vi "SplineParam_Spline_T0_T1.vi"(9 "T1":dbl, 10 "T0":dbl, 11 "inputSPLINE":T5) -> (0 "error out":errorcluster, 3 "outputPOSEwCURVATURE":T1[](array[typedef]))   [LabVIEW 2019, in "Trajectory_Library.lvlib"]
doc: "Parameterizes the spline. This method breaks up the spline into various arcs until their dx, dy, and dtheta are within specific tolerances.\n\nParameters:\n - InputSpline - The spline to parameterize.\n - T0 - Starting internal spline parameter. It is recommended to use 0.0.\n - T1 - Ending internal spline parameter. It is recommended to use 1.0.\n\nReturns:\n - OutputPoseWCurvature - A list of poses and curvatures that represents various points on the spline.\n - Error Out - Returned error cluster"
uses:
  Trajectory_Library.lvlib
  SPLINE.ctl
  <vilib>/Analysis/Matrix/Datatypes/RealMatrix.ctl
  POSEwCURVATURE.ctl
  POSE2D.ctl
  TRANSLATION2D.ctl
  ROTATION2D.ctl
  PARAM_STACK.ctl
  PARAM_STACK_ITEM.ctl
  <vilib>/Analysis/Matrix/NI_Matrix.lvlib
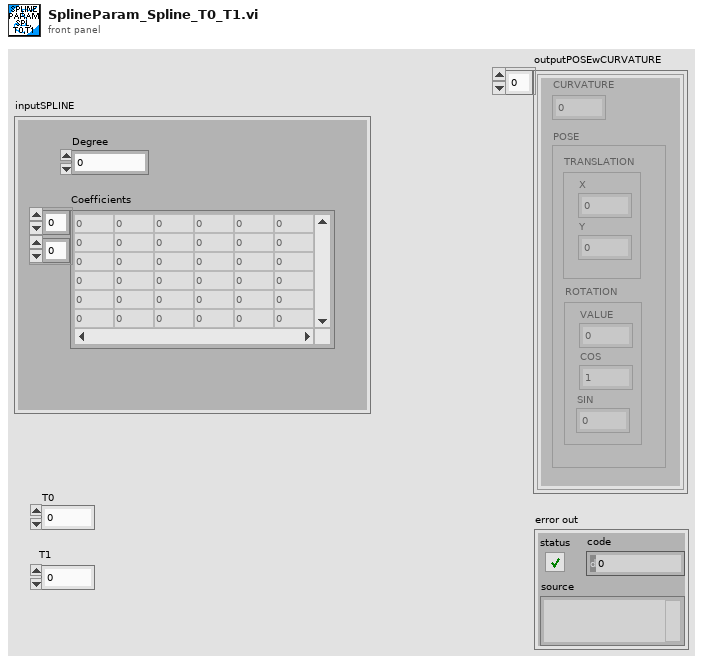
[diagram p1: front panel]
types:
  T1 = typedef "Trajectory_Library.lvlib/POSEwCURVATURE.ctl" = cluster{"CURVATURE":dbl, "POSE":T2}
  T2 = typedef "Trajectory_Library.lvlib/POSE2D.ctl" = cluster{"TRANSLATION":T3, "ROTATION":T4}
  T3 = typedef "Trajectory_Library.lvlib/TRANSLATION2D.ctl" = cluster{"X":dbl, "Y":dbl}
  T4 = typedef "Trajectory_Library.lvlib/ROTATION2D.ctl" = cluster{"VALUE":dbl, "COS":dbl, "SIN":dbl}
  T5 = typedef "Trajectory_Library.lvlib/SPLINE.ctl" = cluster{"Degree":i32, "Coefficients":T6}
  T6 = typedef "NI_Matrix.lvlib/RealMatrix.ctl" = dbl[][]
  T7 = typedef "Trajectory_Library.lvlib/PARAM_STACK.ctl" = cluster{"StackItems":i32, "Stack":T8[]}
  T8 = typedef "Trajectory_Library.lvlib/PARAM_STACK_ITEM.ctl" = cluster{"T0":dbl, "T1":dbl}
  T9 = typedef "Trajectory_Library.lvlib/TWIST2D.ctl" = cluster{"dX":dbl, "dY":dbl, "dTHETA":dbl}
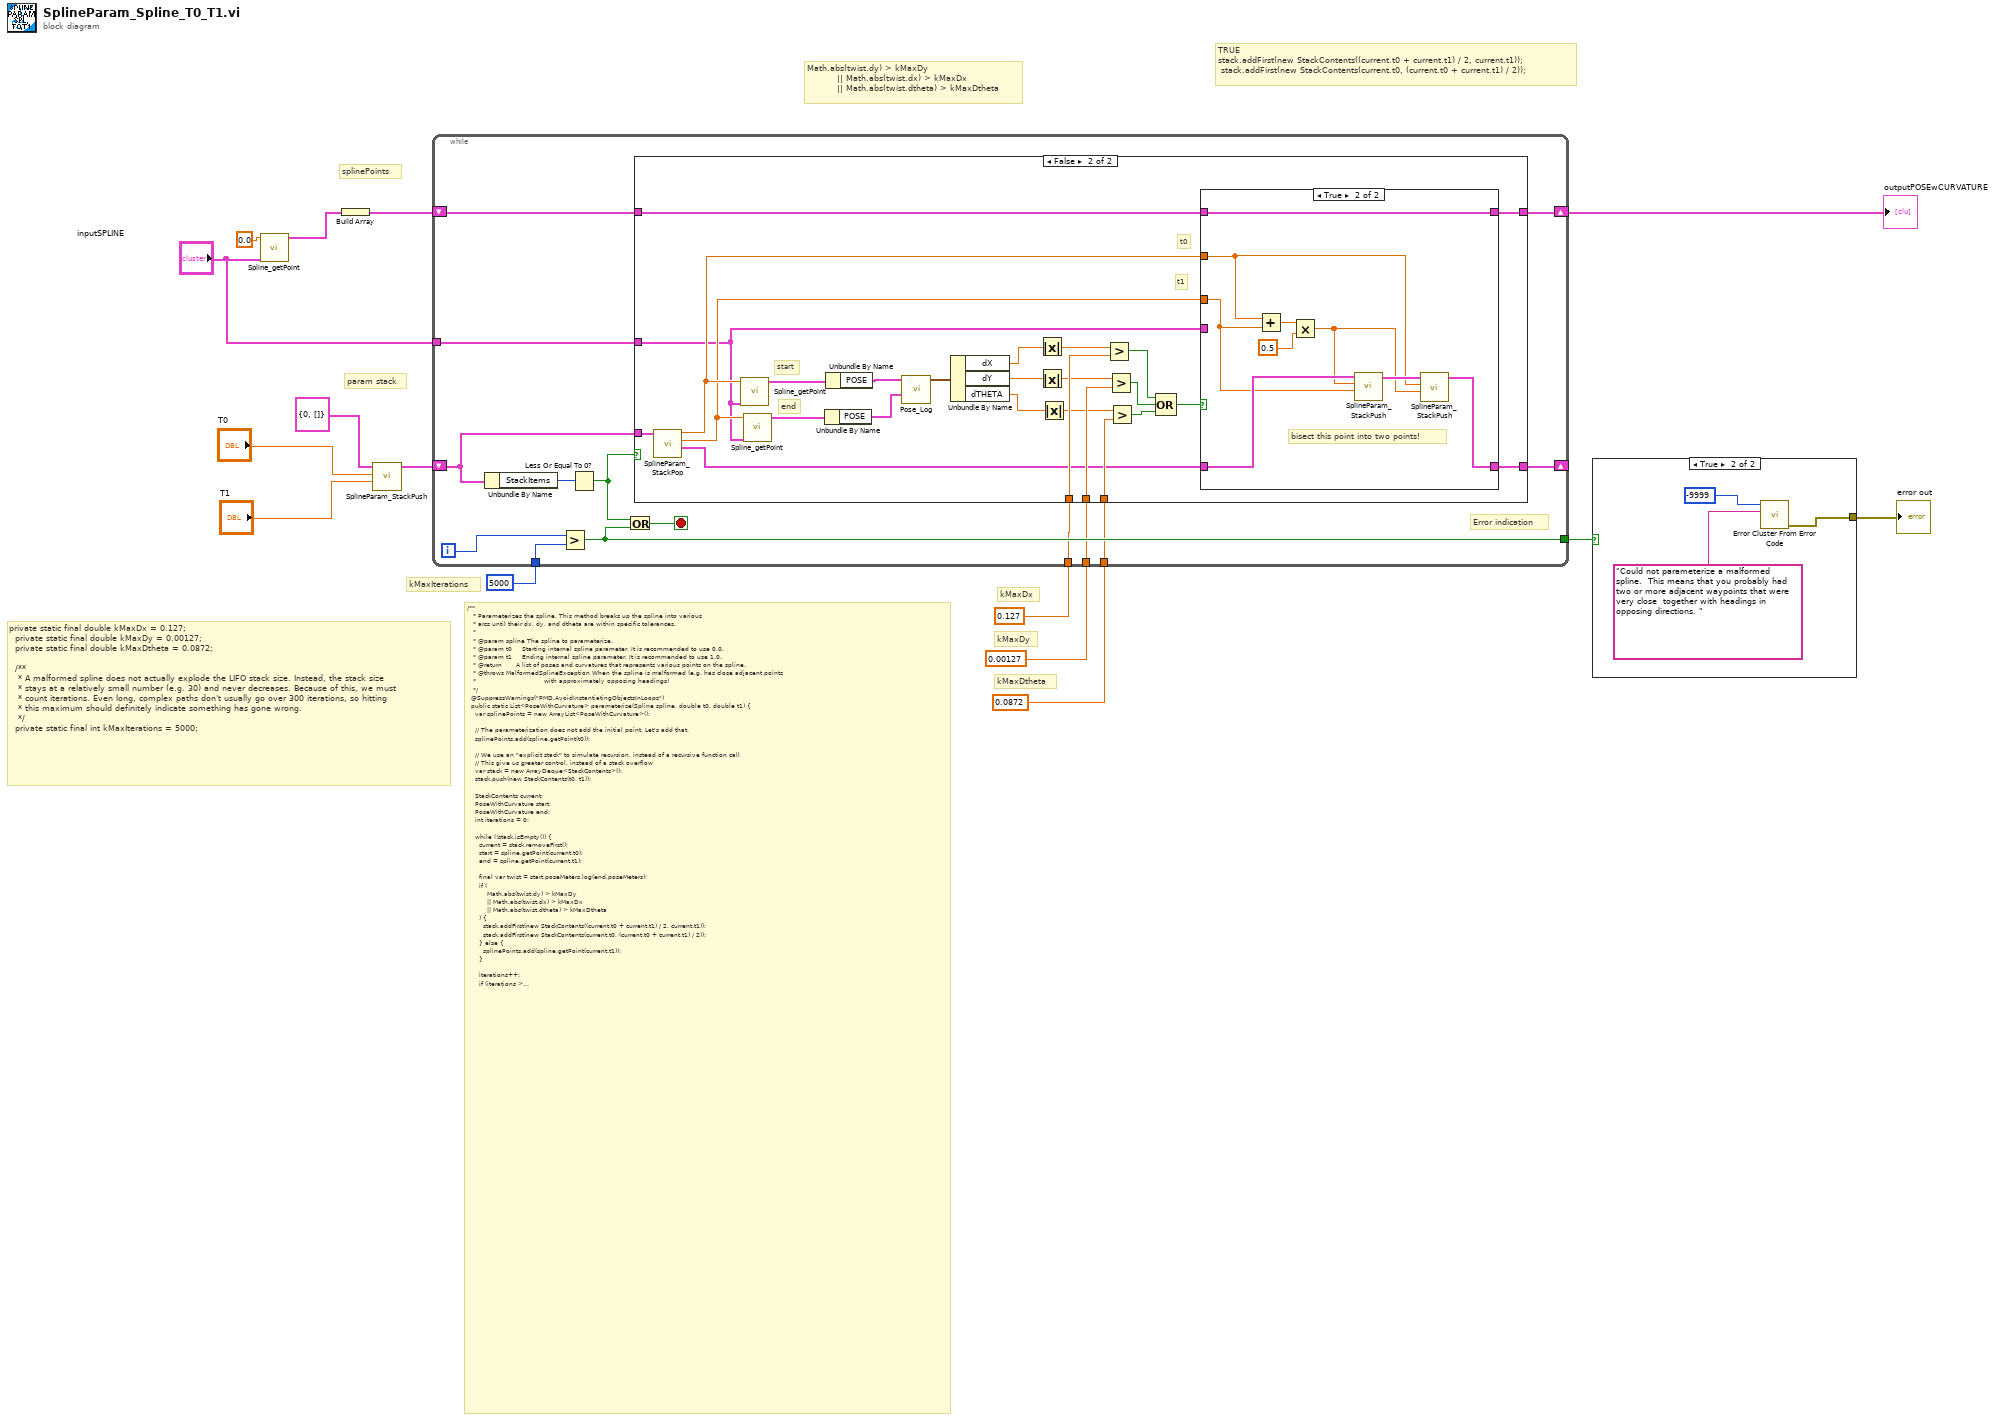
[diagram p0: block diagram]
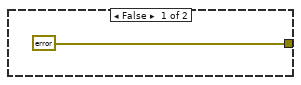
[diagram p2: hidden frame]
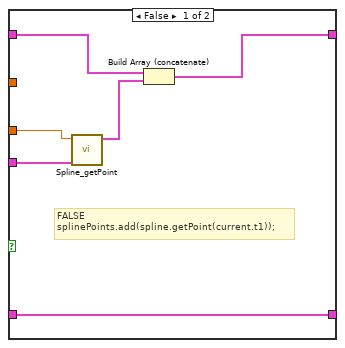
[diagram p4: hidden frame]
diagram:
  # "TRUE\nstack.addFirst(new StackContents((current.t0 + current.t1) / 2, current.t1));\n stack.addFirst(new StackContents(current.t0, (current.t0 + current.t1) / 2));"
  # "splinePoints"
  # "Math.abs(twist.dy) > kMaxDy\n          || Math.abs(twist.dx) > kMaxDx\n          || Math.abs(twist.dtheta) > kMaxDtheta"
  # "kMaxIterations"
  # "kMaxDtheta"
  # "kMaxDy"
  # "kMaxDx"
  # "private static final double kMaxDx = 0.127;\n  private static final double kMaxDy = 0.00127;\n  private static final double kMaxDtheta = 0.0872;\n\n  /**\n   * A malformed spline does not actually explode the LIFO stack size. Instead, the stack size\n   * stays at a relatively small number (e.g. 30) and never decreases. Because of this, we must\n   * count iterations. Even long, complex paths don't usually go over 300 iterations, so hitting\n   * this maximum should definitely indicate something has gone wrong.\n   */\n  private static final int kMaxIterations = 5000;"
  # "param stack"
  # "/**\n   * Parameterizes the spline. This method breaks up the spline into various\n   * arcs until their dx, dy, and dtheta are within specific tolerances.\n   *\n   * @param spline The spline to parameterize.\n   * @param t0     Starting internal spline parameter. It is recommended to use 0.0.\n   * @param t1     Ending internal spline parameter. It is recommended to use 1.0.\n   * @return       A list of poses and curvatures that represents various points on the spline.\n   * @throws MalformedSplineException When the spline is malformed (e.g. has close adjacent points\n   *                                  with approximately opposing headings)\n   */\n  @SuppressWarnings(\"PMD.AvoidInstantiatingObjectsInLoops\")\n  public static List<PoseWithCurvature> parameterize(Spline spline, double t0, double t1) {\n    var splinePoints = new ArrayList<PoseWithCurvature>();\n\n    // The parameterization does not add the initial point. Let's add that.\n    splinePoints.add(spline.getPoint(t0));\n\n    // We use an \"explicit stack\" to simulate recursion, instead of a recursive function call\n    // This give us greater control, instead of a stack overflow\n    var stack = new ArrayDeque<StackContents>();\n    stack.push(new StackContents(t0, t1));\n\n    StackContents current;\n    PoseWithCurvature start;\n    PoseWithCurvature end;\n    int iterations = 0;\n\n    while (!stack.isEmpty()) {\n      current = stack.removeFirst();\n      start = spline.getPoint(current.t0);\n      end = spline.getPoint(current.t1);\n\n      final var twist = start.poseMeters.log(end.poseMeters);\n      if (\n          Math.abs(twist.dy) > kMaxDy\n          || Math.abs(twist.dx) > kMaxDx\n          || Math.abs(twist.dtheta) > kMaxDtheta\n      ) {\n        stack.addFirst(new StackContents((current.t0 + current.t1) / 2, current.t1));\n        stack.addFirst(new StackContents(current.t0, (current.t0 + current.t1) / 2));\n      } else {\n        splinePoints.add(spline.getPoint(current.t1));\n      }\n\n      iterations++;\n      if (iterations >= kMaxIterations) {\n        throw new MalformedSplineException(\n          \"Could not parameterize a malformed spline. \"\n          + \"This means that you probably had two or more adjacent waypoints that were very close \"\n          + \"together with headings in opposing directions.\"\n        );\n      }\n    }\n\n    return splinePoints;\n  }\n}"
  n1 = call "Spline_getPoint.vi"("inputSPLINE"="inputSPLINE", "Time"=0.0) -> ("POSEwCURVATURE"=w1:T1)  [unwired: 9 in]
  n2 = Build Array(w1) -> (w2:T1[])
  n3 = call "SplineParam_StackPush.vi"("T1"="T1", "T0"="T0", "InputStack"=T7 {"StackItems"=0, "Stack"=[]} ("PARAM_STACK")) -> ("OutputStack"=w11:T7)  [unwired: 8 in]
  n4 = while {
    shift-right: [w27] -> _
    shift-left: w11 -> [w29]
    tunnel: "inputSPLINE" -> [w28]
    tunnel: 5000 -> [w24]
    tunnel: [w23] -> w4
    tunnel: 0.127 -> [w22]
    tunnel: 0.00127 -> [w21]
    tunnel: 0.0872 -> [w20]
    shift-right: [w16] -> w5
    shift-left: w2 -> [w17]
    i -> [w25]
    stop <- w26 stop-if-true
    # "Error indication"
    n5 = Unbundle By Name(w29) -> ("StackItems"=w19:i32)
    n6 = Greater?(x=w25, y=w24) -> (0:w23:bool)
    n7 = Less Or Equal To 0?(x=w19) -> (x <= 0?=w18:bool)
    n8 = Or(x=w18, y=w23) -> (x .or. y?=w26:bool)
    n9 = case shown="False" w18 {
      tunnel: w29 -> [w30 w57]
      tunnel: w28 -> [_ w32]
      tunnel: [w30 w56] -> w27
      tunnel: w22 -> [_ w55]
      tunnel: w21 -> [_ w54]
      tunnel: w20 -> [_ w53]
      tunnel: w17 -> [w31 w34]
      tunnel: [w31 w33] -> w16
      frame True {
      }
      frame False {
        # "t1"
        # "t0"
        # "end"
        # "start"
        n10 = call "SplineParam_StackPop.vi"("InputStack"=w57) -> ("outputStack"=w37:T7, "T1"=w35:dbl, "T0"=w36:dbl)  [unwired: 8 in]
        n11 = call "Spline_getPoint.vi"("inputSPLINE"=w32, "Time"=w36) -> ("POSEwCURVATURE"=w52:T1)  [unwired: 9 in]
        n12 = call "Spline_getPoint.vi"("inputSPLINE"=w32, "Time"=w35) -> ("POSEwCURVATURE"=w50:T1)  [unwired: 9 in]
        n13 = Unbundle By Name(w50) -> ("POSE"=w49:T2)
        n14 = Unbundle By Name(w52) -> ("POSE"=w51:T2)
        n15 = call "Pose_Log.vi"("end POSE"=w49, "in POSE"=w51) -> ("out TWIST"=w48:T9)  [unwired: 9 in]
        n16 = Unbundle By Name(w48) -> ("dX"=w47:dbl, "dY"=w46:dbl, "dTHETA"=w45:dbl)
        n17 = Absolute Value(x=w47) -> (abs(x)=w44:dbl)
        n18 = Absolute Value(x=w46) -> (abs(x)=w43:dbl)
        n19 = Absolute Value(x=w45) -> (abs(x)=w42:dbl)
        n20 = Greater?(x=w44, y=w55) -> (0:w39:bool)
        n21 = Greater?(x=w43, y=w54) -> (0:w40:bool)
        n22 = Greater?(x=w42, y=w53) -> (0:w41:bool)
        n23 = Compound Arithmetic op=OR(w39, w40, w41) -> (w38:bool)
        n24 = case shown="True" w38 {
          tunnel: w37 -> [w63 w72]
          tunnel: [w63 w70] -> w56
          tunnel: w36 -> [_ w66]
          tunnel: w35 -> [w61 w67]
          tunnel: w34 -> [w62 w64]
          tunnel: [w58 w64] -> w33
          tunnel: w32 -> [w60 _]
          frame False {
            # "FALSE\nsplinePoints.add(spline.getPoint(current.t1));"
            n25 = call "Spline_getPoint.vi"("inputSPLINE"=w60, "Time"=w61) -> ("POSEwCURVATURE"=w59:T1)  [unwired: 9 in]
            n26 = Build Array (concatenate)(w62, w59) -> (w58:T1[])
          }
          frame True {
            # "bisect this point into two points!"
            n27 = Add(x=w66, y=w67) -> (x+y=w69:dbl)
            n28 = Multiply(x=w69, y=0.5) -> (x*y=w65:dbl)
            n29 = call "SplineParam_StackPush.vi"("T1"=w67, "T0"=w65, "InputStack"=w72) -> ("OutputStack"=w71:T7)  [unwired: 8 in]
            n30 = call "SplineParam_StackPush.vi"("T1"=w65, "T0"=w66, "InputStack"=w71) -> ("OutputStack"=w70:T7)  [unwired: 8 in]
          }
        }
      }
    }
  }
  "outputPOSEwCURVATURE" <- w5
  n31 = case shown="True" w4 {
    tunnel: [errorcluster {"status"=FALSE, "code"=0, "source"=""} ("error out") w74] -> w3
    frame False {
    }
    frame True {
      n32 = call <vilib>:"Error Cluster From Error Code.vi"("error message (\"\")"="Could not parameterize a malformed spline.  This means that you probably had two or more adjacent waypoints that were very close  together with headings in opposing directions. " ("error message (\"\")"), "error code (0)"=-9999) -> ("error out"=w74:errorcluster)  [unwired: 7 in]
    }
  }
  "error out" <- w3
